vi "GUI.vi"() -> ()   [LabVIEW 2021]
uses:
  <vilib>/numeric/Random Number (Range) U64.vi
  <vilib>/numeric/sub_Random U32.vi
  <vilib>/Instr/_visa.llb/VISA Configure Serial Port (Instr).vi
panel:
  out "start sim":bool
  out "Time has Elapsed":bool
  out "Time":dbl
  out "Logging":bool caption="Time has Elapsed"
  in  "PWM":i16(slide)=1410 min=1300 max=1410 scale=1155.0..1384.0
  out "Mode":string
  in  "Mode":bool
  out "O":dbl
  out "T":dbl
  out "D":dbl
  out "I":dbl
  out "P":dbl
  out "F":dbl
  out "S":dbl
  in  "Stop Button":bool
  out "TS":dbl(slide) scale=0.0..100.0
  out "KD":dbl(slide) scale=0.0..100.0
  out "KI":dbl(slide) scale=0.0..50.0
  out "KP":dbl(slide) scale=0.0..10.0
  in  "COM Port":refnum<visa-resource-name>
  in  "Save Result":path
  out "Output PID":dbl(graph)
  out "Tacho Generator":dbl(knob) scale=0.0..1023.0
  out "SetPoint":dbl(knob) scale=0.0..1023.0
  out "Respon PID":dynamicdata(graph)
  # "ALIM SATRIA FI'I WIJAYA KUSUMA (21/483503/SV/20304)"
  # "KENDALI KECEPATAN MOTOR DC"
  # "ILHAM DWI CAHYO (21/483417/SV/20218)"
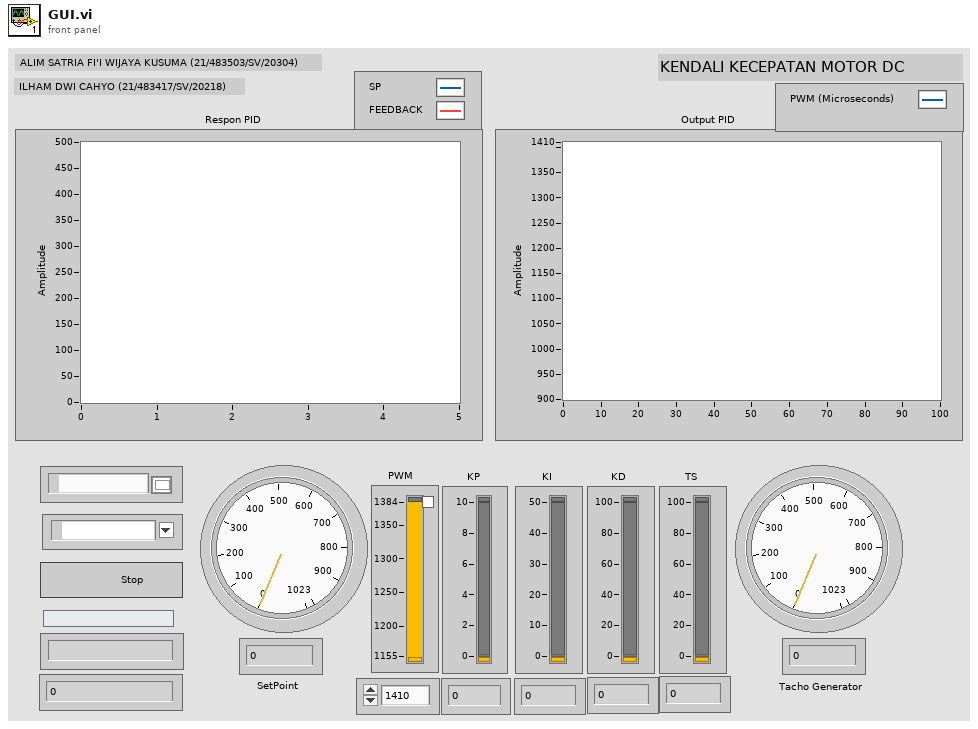
[diagram p1: front panel]
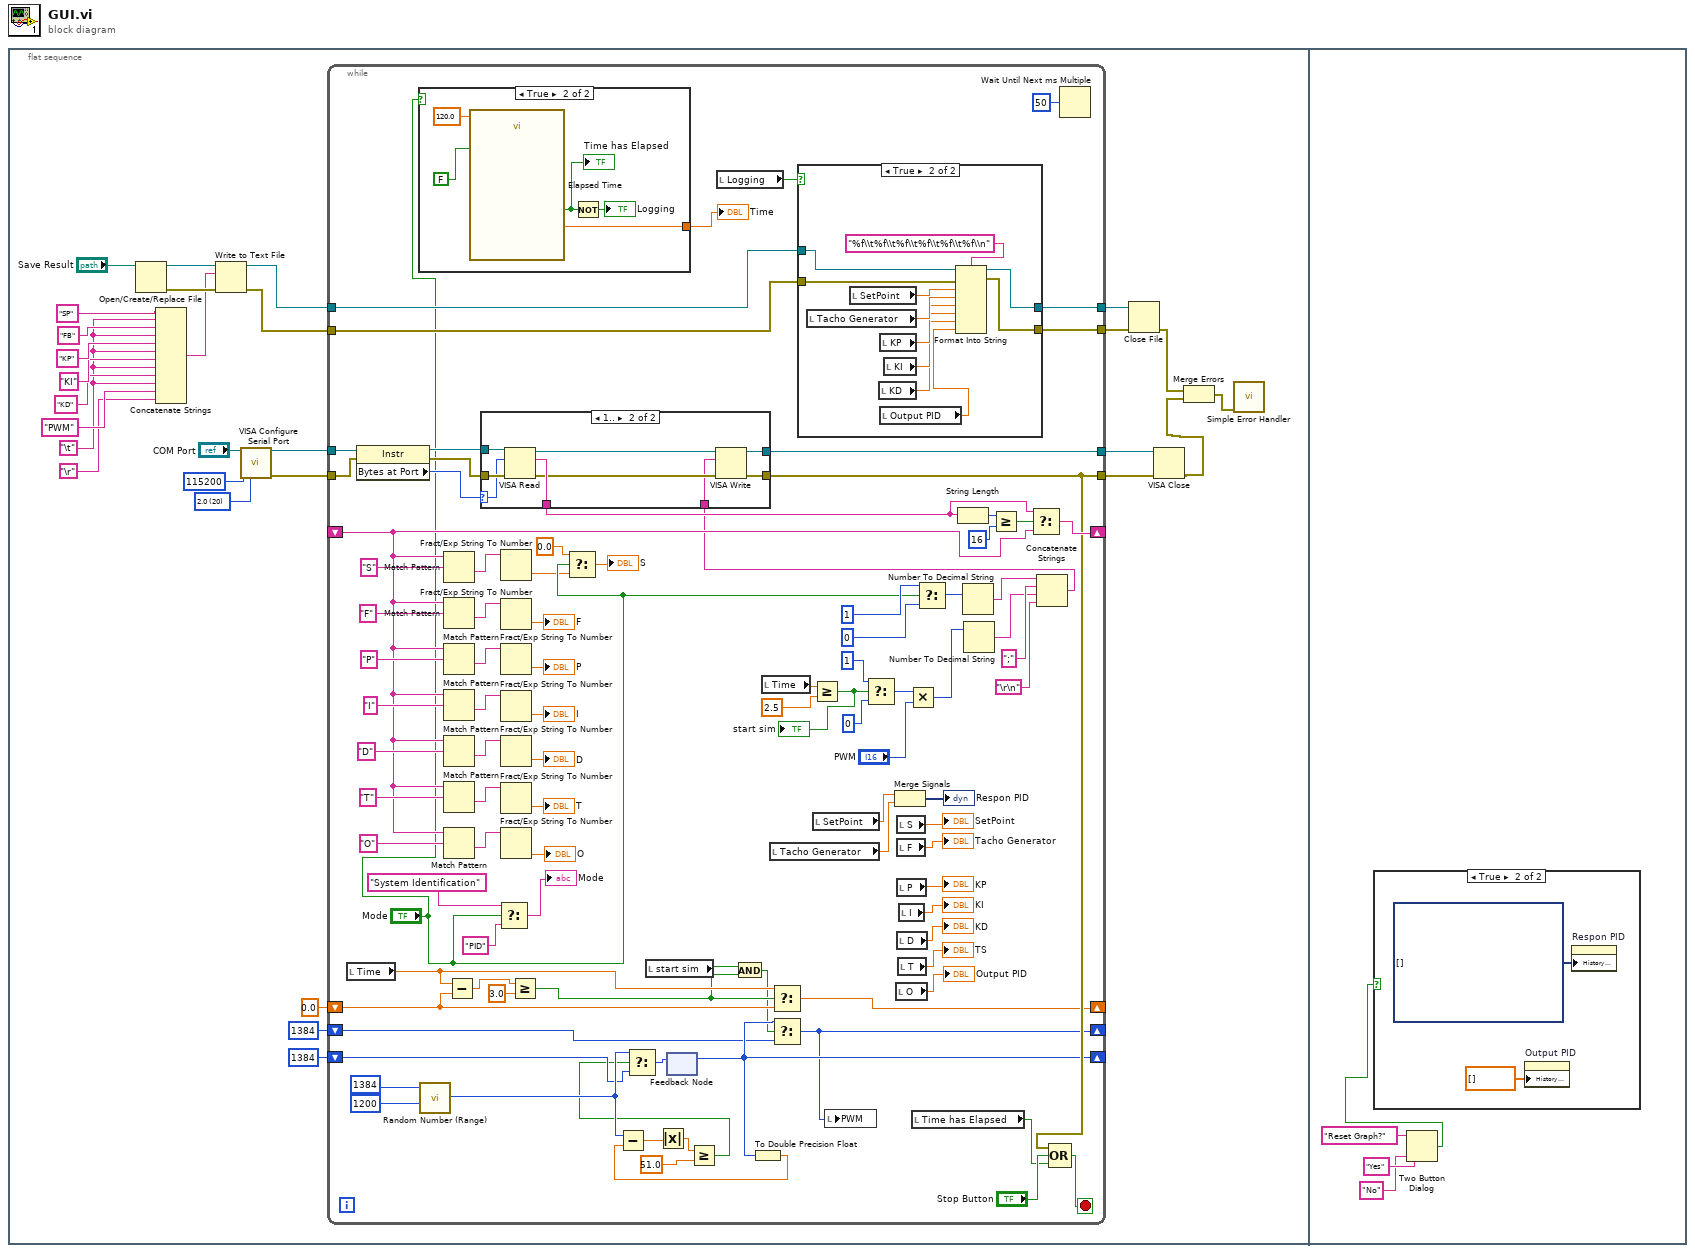
[diagram p0: block diagram]
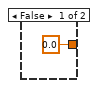
[diagram p2: hidden frame]
diagram:
  n1 = flat-sequence {
    frame #0 {
      w1 = u16 20 items=["1.0"=10, "1.5"=15, "2.0"=20] ("stop bits (10: 1 bit)")
      w12 = "\t"
      n2 = Open/Create/Replace File(file path (use dialog)="Save Result") -> (refnum out=w24:refnum<file>, error out=w25:errorcluster)  [unwired: 5 in, 1 out]
      n3 = Concatenate Strings("SP", w12, "FB" ("string"), w12, "KP" ("string"), w12, "KI" ("string"), w12, "KD" ("string"), w12, "PWM", "\r") -> (w19:string)
      n4 = Write to Text File(file (use dialog)=w24, text=w19, error in=w25) -> (refnum out=w23:refnum<file>, error out=w22:errorcluster)  [unwired: 1 in, 1 out]
      n5 = call-poly "VISA Configure Serial Port"("VISA resource name"="COM Port", "baud rate (9600)"=u32 115200, "stop bits (10: 1 bit)"=w1) -> ("VISA resource name out"=w29:refnum<visa-resource-name>, "error out"=w28:errorcluster)  [unwired: 11 in]
      n6 = while {
        tunnel: w29 -> [w85]
        tunnel: w28 -> [w81]
        tunnel: [w82] -> w10
        tunnel: [w76] -> w9
        tunnel: w23 -> [w95]
        tunnel: w22 -> [w94]
        tunnel: [w93] -> w21
        tunnel: [w92] -> w20
        shift-right: [w88] -> _
        shift-left: _ -> [w87]
        shift-right: [w35] -> _
        shift-left: u64 1384 ("number") -> [w37]
        shift-right: [w42] -> _
        shift-left: 0.0 ("Time") -> [w38]
        shift-right: [w33] -> _
        shift-left: u64 1384 ("number") -> [w34]
        stop <- w126 stop-if-true
        n7 = local read "Time"() -> (w39:dbl)
        n8 = property class="Instr"(reference=w85, error in=w81) -> (reference out=w84:refnum<visa-resource-name>, error out=w83:errorcluster, "Bytes at Port"=w125:u32)
        n9 = case shown="True" "Mode" {
          tunnel: [0.0 ("Elapsed Time (s)") w129] -> w65
          frame False {
          }
          frame True {
            n10 = call "Elapsed Time"("Time Target (s)"=120.0, "Auto Reset"=FALSE) -> ("Elapsed Time (s)"=w129:dbl, "Time has Elapsed"=w132:bool)  [unwired: 10 in, 6 out]
            "Time has Elapsed" <- w132
            n11 = Not(x=w132) -> (.not. x?=→"Logging":bool)
          }
        }
        "Time" <- w65
        n12 = call-poly <vilib>:"Random Number (Range).vi"("lower bound (0)"=u64 1200, "upper bound (100)"=u64 1384) -> ("number"=w49:u64)  [unwired: 9 in]
        n13 = Match Pattern(string=w87, regular expression="S") -> (after substring=w117:string)  [unwired: 1 in, 3 out]
        n14 = Match Pattern(string=w87, regular expression="F") -> (after substring=w116:string)  [unwired: 1 in, 3 out]
        n15 = Match Pattern(string=w87, regular expression="P") -> (after substring=w115:string)  [unwired: 1 in, 3 out]
        n16 = Match Pattern(string=w87, regular expression="I") -> (after substring=w114:string)  [unwired: 1 in, 3 out]
        n17 = Match Pattern(string=w87, regular expression="D") -> (after substring=w113:string)  [unwired: 1 in, 3 out]
        n18 = Match Pattern(string=w87, regular expression="T") -> (after substring=w112:string)  [unwired: 1 in, 3 out]
        n19 = Match Pattern(string=w87, regular expression="O") -> (after substring=w111:string)  [unwired: 1 in, 3 out]
        n20 = Subtract(x=w39, y=w38) -> (x-y=w40:dbl)
        n21 = Select(t="System Identification", s="Mode", f="PID") -> (s? t:f=→"Mode":string)
        n22 = Fract/Exp String To Number(string=w117) -> (number=w54:dbl)  [unwired: 3 in, 1 out]
        n23 = Fract/Exp String To Number(string=w116) -> (number=→"F":dbl)  [unwired: 3 in, 1 out]
        n24 = Fract/Exp String To Number(string=w115) -> (number=→"P":dbl)  [unwired: 3 in, 1 out]
        n25 = Fract/Exp String To Number(string=w114) -> (number=→"I":dbl)  [unwired: 3 in, 1 out]
        n26 = Fract/Exp String To Number(string=w113) -> (number=→"D":dbl)  [unwired: 3 in, 1 out]
        n27 = Fract/Exp String To Number(string=w112) -> (number=→"T":dbl)  [unwired: 3 in, 1 out]
        n28 = Fract/Exp String To Number(string=w111) -> (number=→"O":dbl)  [unwired: 3 in, 1 out]
        n29 = Greater Or Equal?(x=w40, y=3.0) -> (x >= y?=w31:bool)
        n30 = Select(t=0.0, s="Mode", f=w54) -> (s? t:f=→"S":dbl)
        n31 = local read "start sim"() -> (w32:bool)
        n32 = feedback #1() -> (w35:u64)  [unwired: 1 in]
        n33 = local read "Logging"() -> (w66:bool)
        n34 = And(x=w32, y=w31) -> (x .and. y?=w30:bool)
        n35 = To Double Precision Float(number=w35) -> (double precision float=w45:dbl)
        n36 = Subtract(x=w49, y=w45) -> (x-y=w47:dbl)
        n37 = Absolute Value(x=w47) -> (abs(x)=w48:dbl)
        n38 = Greater Or Equal?(x=w48, y=51.0) -> (x >= y?=w36:bool)
        n39 = Select(t=w49, s=w36, f=w37) -> (s? t:f=w46:u64)
        n40 = feedback-in #1(w46) -> ()
        n41 = local read "Time"() -> (w63:dbl)
        n42 = local read "Tacho Generator"() -> (w103:dbl)
        n43 = Select(t=w39, s=w31, f=w38) -> (s? t:f=w42:dbl)
        n44 = Select(t=w35, s=w30, f=w34) -> (s? t:f=w33:u64)
        n45 = case shown="True" w66 {
          tunnel: w95 -> [w134 w145]
          tunnel: w94 -> [w133 w144]
          tunnel: [w134 w143] -> w93
          tunnel: [w133 w142] -> w92
          frame False {
          }
          frame True {
            n46 = local read "Tacho Generator"() -> (w140:dbl)
            n47 = local read "SetPoint"() -> (w141:dbl)
            n48 = local read "KD"() -> (w136:dbl)
            n49 = local read "KP"() -> (w138:dbl)
            n50 = local read "Output PID"() -> (w135:dbl)
            n51 = local read "KI"() -> (w137:dbl)
            n52 = Format Into String(format string="%f\\t%f\\t%f\\t%f\\t%f\\t%f\\n", initial string=w145, error in=w144, w141, w140, w138, w137, w136, w135) -> (resulting string=w143:refnum<file>, error out=w142:errorcluster)
          }
        }
        n53 = Greater Or Equal?(x=w63, y=2.5) -> (x >= y?=w61:bool)
        "start sim" <- w61
        n54 = local read "SetPoint"() -> (w104:dbl)
        n55 = local write "PWM"(w33) -> ()
        n56 = Select(t=i16 1, s=w61, f=i16 0) -> (s? t:f=w58:i16)
        n57 = Merge Signals(w104, w103) -> (→"Respon PID":dynamicdata)
        n58 = local read "O"() -> (→"Output PID":dbl)
        n59 = local read "S"() -> (→"SetPoint":dbl)
        n60 = local read "F"() -> (→"Tacho Generator":dbl)
        n61 = local read "P"() -> (→"KP":dbl)
        n62 = local read "D"() -> (→"KD":dbl)
        n63 = local read "T"() -> (→"TS":dbl)
        n64 = local read "I"() -> (→"KI":dbl)
        n65 = Multiply(x=w58, y="PWM") -> (x*y=w56:i16)
        n66 = local read "Time has Elapsed"() -> (w64:bool)
        n67 = Select(t=1, s="Mode", f=0) -> (s? t:f=w68:i32)
        n68 = Number To Decimal String(number=w68) -> (decimal integer string=w72:string)  [unwired: 1 in]
        n69 = Number To Decimal String(number=w56) -> (decimal integer string=w71:string)  [unwired: 1 in]
        n70 = Concatenate Strings(w72, ";", w71, "\r\n") -> (w75:string)
        n71 = case shown="1.." w125 {
          selector: w125 -> [_ w153]
          tunnel: w84 -> [w147 w156]
          tunnel: [w147 w150] -> w82
          tunnel: w83 -> [w146 w155]
          tunnel: [w146 w149] -> w76
          tunnel: [_ w154] -> w86
          tunnel: w75 -> [_ w148]
          frame 0, Default {
          }
          frame 1.. {
            n72 = VISA Read(VISA resource name=w156, byte count=w153, error in (no error)=w155) -> (VISA resource name out=w152:refnum<visa-resource-name>, read buffer=w154:string, error out=w151:errorcluster)  [unwired: 1 out]
            n73 = VISA Write(VISA resource name=w152, write buffer=w148, error in (no error)=w151) -> (VISA resource name out=w150:refnum<visa-resource-name>, error out=w149:errorcluster)  [unwired: 1 out]
          }
        }
        n74 = String Length(string=w86) -> (length=w91:i32)
        n75 = Greater Or Equal?(x=w91, y=16) -> (x >= y?=w89:bool)
        n76 = Select(t=w86, s=w89, f=w87) -> (s? t:f=w88:string)
        n77 = Compound Arithmetic op=OR(w76, "Stop Button", w64) -> (w126:bool)
        n78 = Wait Until Next ms Multiple(millisecond multiple=u32 50) -> ()  [unwired: 1 out]
      }
      n79 = Close File(refnum=w21, error in=w20) -> (error out=w8:errorcluster)  [unwired: 1 out]
      n80 = VISA Close(VISA resource name=w10, error in (no error)=w9) -> (error out=w7:errorcluster)
      n81 = Merge Errors(w8, w7) -> (w6:errorcluster)
      n82 = call <vilib>:"Simple Error Handler.vi"("error in (no error)"=w6) -> ()  [unwired: 4 in, 5 out]
    }
    frame #1 {
      n83 = Two Button Dialog(message="Reset Graph?", 1:"No" ("F button name (\"Cancel\")"), 2:"Yes" ("T button name (\"OK\")")) -> (T button?=w157:bool)
      n84 = case shown="True" w157 {
        frame False {
        }
        frame True {
          n85 = property on="Output PID" class="WFChart (strict)"("History Data"=dbl[] []) -> ()  [unwired: 2 in, 2 out]
          n86 = property on="Respon PID" class="WFChart (strict)"("History Data"=dynamicdata[] []) -> ()  [unwired: 2 in, 2 out]
        }
      }
    }
  }
